vi "ProducerConsummerLoopGen.vi"() -> ()   [LabVIEW 2019, in "BaseDevice.lvclass"]
uses:
  Programmes LabView/LabScanV1A/DevicesClass/BaseDevice/BaseDevice.lvclass
  Programmes LabView/LabScanV1A/Experiment Class/Experiment.lvclass
  Programmes LabView/LabScanV1A/DevicesClass/BaseDevice/BaseDevice.lvclass/BaseDevice.ctl
panel:
  in  "AssignDat":bool
  in  "Stop":bool
  out "ErrOut":errorcluster caption="sortie d'erreur"
  out "Experiment.lvclassOut":refnum<class "Experiment.lvclass">
  out "DeviceCtrls":T1(array[cluster])
  in  "SrcData":enum16{""}(ring) caption="Data Source"
  in  "TargetInstr":enum16{""}(ring) caption="Source Instrument"
  in  "SrcInstr":enum16{""}(ring) caption="Target Instrument"
  in  "ErrorIn (NoErr)":errorcluster caption="entrée d'erreur (pas d'erreur)"
  in  "Experiment.lvclass":refnum<class "Experiment.lvclass">
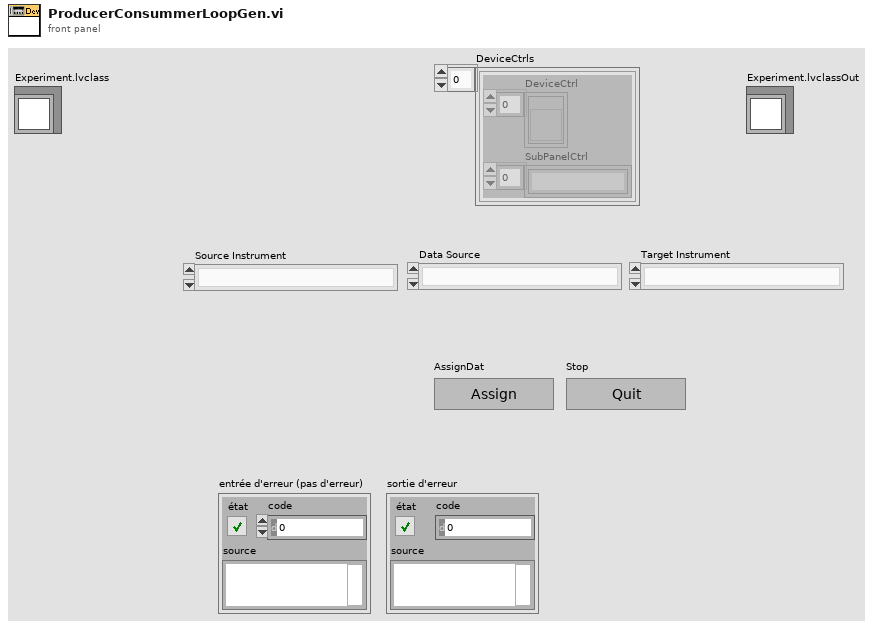
[diagram p1: front panel]
types:
  T1 = cluster{"DeviceCtrl":refnum<vi>[], "SubPanelCtrl":string[]}[]
  T2 = cluster{"Message":string, "Data":variant, "Code":i32}
  T3 = cluster{"DeviceCtrl":refnum<vi>[], "SubPanelCtrl":string[]}
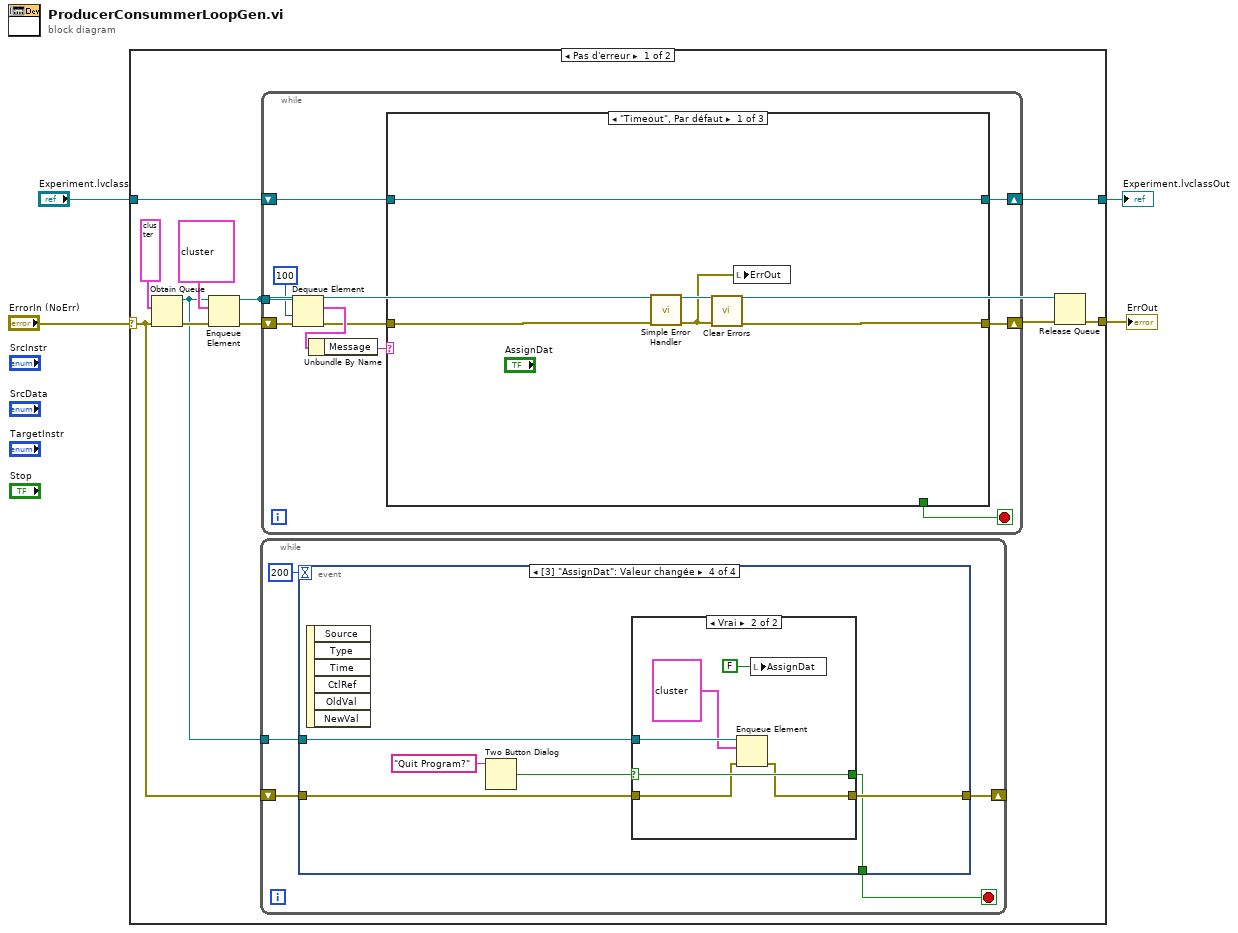
[diagram p0: block diagram]
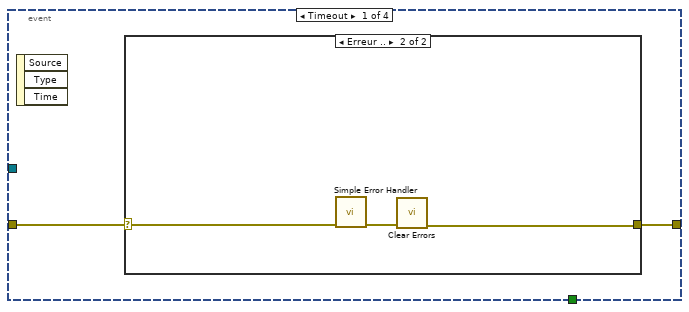
[diagram p2: hidden frame]
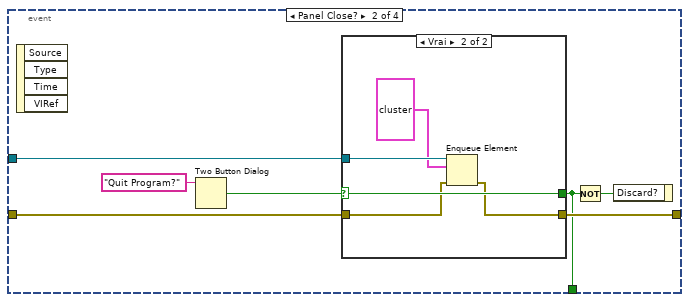
[diagram p4: hidden frame]
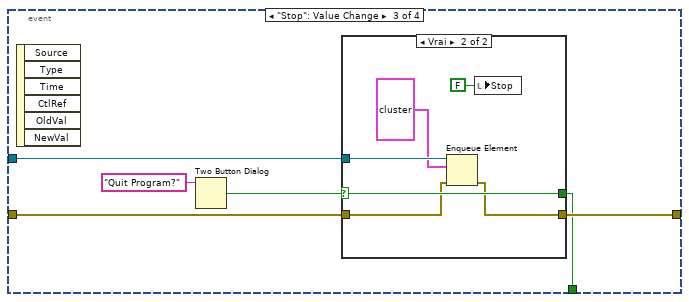
[diagram p6: hidden frame]
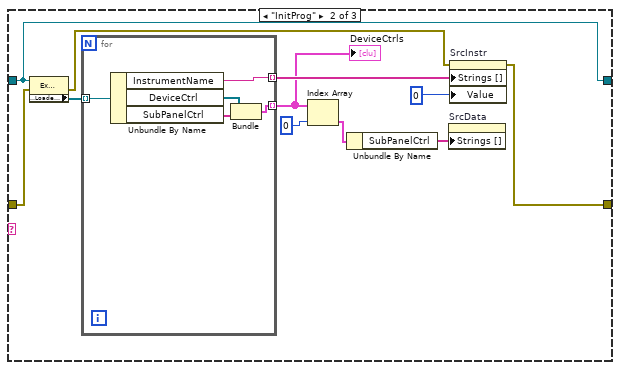
[diagram p9: hidden frame]
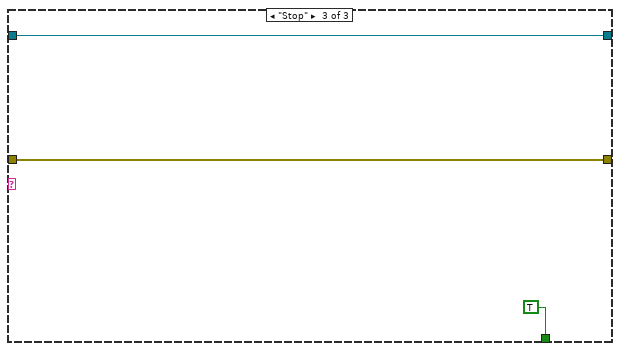
[diagram p10: hidden frame]
diagram:
  n1 = case shown="Pas d'erreur" "ErrorIn (NoErr)" {
    selector: "ErrorIn (NoErr)" -> [w10 w102]
    tunnel: "Experiment.lvclass" -> [w15 w103]
    tunnel: [w7 w103] -> w2
    tunnel: [w5 w102] -> w1
    frame No Error {
      n2 = Obtain Queue(element data type=T2 {"Message"="", "Data"=variant, "Code"=0} ("élément"), error in (no error)=w10) -> (queue out=w9:refnum<queue>, error out=w13:errorcluster)  [unwired: 3 in, 1 out]
      n3 = Enqueue Element(queue=w9, element=T2 {"Message"="InitProg", "Data"=variant, "Code"=0} ("élément"), error in (no error)=w13) -> (queue out=w8:refnum<queue>, error out=w12:errorcluster)  [unwired: 1 in, 1 out]
      n4 = while {
        tunnel: w9 -> [w18]
        shift-right: [w17] -> _
        shift-left: w10 -> [w19]
        stop <- w16 stop-if-true
        n5 = event shown="[3] \"AssignDat\": Valeur changée" {
          selector: _ -> [_ _ _ _]
          dyn-events: _ -> [_ _ _ _]
          timeout: 200 -> [_ _ _ _]
          tunnel: w19 -> [w22 w29 w43 w57]
          tunnel: w18 -> [_ w33 w46 w60]
          tunnel: [w21 w28 w42 w56] -> w17
          tunnel: [_ w27 w41 w55] -> w16
          event Timeout {
            n6 = event-data() -> ()  [unwired: 1 in, 3 out]
            n7 = case shown="Erreur .." w22 {
              selector: w22 -> [w23 w26]
              tunnel: [w23 w24] -> w21
              frame No Error {
              }
              frame Error {
                n8 = call <vilib>:"Simple Error Handler.vi"("error in (no error)"=w26) -> ("error out"=w25:errorcluster)  [unwired: 4 in, 4 out]
                n9 = call <vilib>:"Clear Errors.vi"("error in (no error)"=w25) -> ("error out"=w24:errorcluster)  [unwired: 5 in, 1 out]
              }
            }
          }
          event Panel Close? {
            n10 = event-data() -> ()  [unwired: 1 in, 4 out]
            n11 = Two Button Dialog(message="Quit Program?") -> (T button?=w32:bool)  [unwired: 2 in]
            n12 = case shown="Vrai" w32 {
              selector: w32 -> [w35 w38]
              tunnel: w33 -> [_ w40]
              tunnel: [w35 w38] -> w27
              tunnel: w29 -> [w34 w37]
              tunnel: [w34 w36] -> w28
              frame False {
              }
              frame True {
                n13 = Enqueue Element(queue=w40, element=T2 {"Message"="Stop", "Data"=variant, "Code"=0} ("élément"), error in (no error)=w37) -> (error out=w36:errorcluster)  [unwired: 1 in, 2 out]
              }
            }
            n14 = Not(x=w27) -> (.not. x?=w30:bool)
            n15 = event-data("Discard?"=w30) -> ()  [unwired: 1 in, 1 out]
          }
          event "Stop": Value Change {
            n16 = event-data() -> ()  [unwired: 1 in, 6 out]
            n17 = Two Button Dialog(message="Quit Program?") -> (T button?=w45:bool)  [unwired: 2 in]
            n18 = case shown="Vrai" w45 {
              selector: w45 -> [w48 w52]
              tunnel: w46 -> [_ w54]
              tunnel: [w48 w52] -> w41
              tunnel: w43 -> [w47 w51]
              tunnel: [w47 w50] -> w42
              frame False {
              }
              frame True {
                n19 = Enqueue Element(queue=w54, element=T2 {"Message"="Stop", "Data"=variant, "Code"=0} ("élément"), error in (no error)=w51) -> (error out=w50:errorcluster)  [unwired: 1 in, 2 out]
                n20 = local write "Stop"(FALSE ("Stop")) -> ()
              }
            }
          }
          event "AssignDat": Value Change {
            n21 = event-data() -> ()  [unwired: 1 in, 6 out]
            n22 = Two Button Dialog(message="Quit Program?") -> (T button?=w59:bool)  [unwired: 2 in]
            n23 = case shown="Vrai" w59 {
              selector: w59 -> [w62 w66]
              tunnel: w60 -> [_ w68]
              tunnel: [w62 w66] -> w55
              tunnel: w57 -> [w61 w65]
              tunnel: [w61 w64] -> w56
              frame False {
              }
              frame True {
                n24 = Enqueue Element(queue=w68, element=T2 {"Message"="Assign", "Data"=variant, "Code"=0} ("élément"), error in (no error)=w65) -> (error out=w64:errorcluster)  [unwired: 1 in, 2 out]
                n25 = local write "AssignDat"(FALSE ("Stop")) -> ()
              }
            }
          }
        }
      }
      n26 = while {
        shift-right: [w71] -> w6
        shift-left: w12 -> [w78]
        shift-right: [w72] -> w7
        shift-left: w15 -> [w75]
        tunnel: w8 -> [w73]
        stop <- w70 stop-if-true
        n27 = Dequeue Element(queue=w73, timeout in ms (-1)=100 ("timeout en ms (-1)"), error in (no error)=w78) -> (element=w77:T2, error out=w74:errorcluster)  [unwired: 2 out]
        n28 = Unbundle By Name(w77) -> ("Message"=w76:string)
        n29 = case shown="\"Timeout\", Par défaut" w76 {
          tunnel: w75 -> [w82 w85 w101]
          tunnel: w74 -> [w81 w92 w100]
          tunnel: [w82 w85 w101] -> w72
          tunnel: [w80 w83 w100] -> w71
          tunnel: [_ _ TRUE ("Stop")] -> w70
          frame "Timeout", Default {
            n30 = call <vilib>:"Simple Error Handler.vi"("error in (no error)"=w81) -> ("error out"=w79:errorcluster)  [unwired: 4 in, 4 out]
            n31 = call <vilib>:"Clear Errors.vi"("error in (no error)"=w79) -> ("error out"=w80:errorcluster)  [unwired: 5 in, 1 out]
            n32 = local write "ErrOut"(w79) -> ()
          }
          frame "InitProg" {
            n33 = property class="Experiment.lvclass"(reference=w85, error in=w92) -> (error out=w84:errorcluster, "Accessor:LoadedInst"=w93:refnum<class "BaseDevice.lvclass">[])  [unwired: 1 out]
            n34 = for {
              tunnel: w93 -> [w98] mode=indexing
              tunnel: [w97] -> w91 mode=indexing
              tunnel: [w94] -> w86 mode=indexing
              n35 = Unbundle By Name(w98) -> ("InstrumentName"=w97:string, "DeviceCtrl"=w96:refnum<vi>[], "SubPanelCtrl"=w95:string[])
              n36 = Bundle("DeviceCtrl"=w96, "SubPanelCtrl"=w95) -> (w94:T3)  [unwired: 1 in]
            }
            "DeviceCtrls" <- w86
            n37 = Index Array(array=w86, index=0 ("indice (ligne)")) -> (element=w88:T3)
            n38 = Unbundle By Name(w88) -> ("SubPanelCtrl"=w87:string[])
            n39 = property on="SrcData" class="Énum (strict)"("Strings []"=w87) -> ()  [unwired: 2 in, 2 out]
            n40 = property on="SrcInstr" class="Énum (strict)"(error in=w84, "Strings []"=w91, "Value"=u16 0 ("indice (ligne)")) -> (error out=w83:errorcluster)  [unwired: 1 in, 1 out]
          }
          frame "Stop" {
          }
        }
      }
      n41 = Release Queue(queue=w8, error in (no error)=w6) -> (error out=w5:errorcluster)  [unwired: 1 in, 2 out]
    }
    frame Error {
    }
  }
  "Experiment.lvclassOut" <- w2
  "ErrOut" <- w1
